vi "Read Status.vi"(6 "Selector":T1, 8 "error in":errorcluster, 11 "MiniIO in":refnum<class "MiniIO.lvclass">) -> (0 "error out":errorcluster, 3 "MiniIO out":refnum<class "MiniIO.lvclass">)   [LabVIEW 2018, in "MiniIO.lvlib" / "MiniIO.lvclass"]
uses:
  MiniIO.lvclass
  PPLs/PLC/Parent/PLC.lvlibp/Custom Controls/Selector.ctl
  PPLs/PLC/Parent/PLC.lvlibp/PLC.lvclass
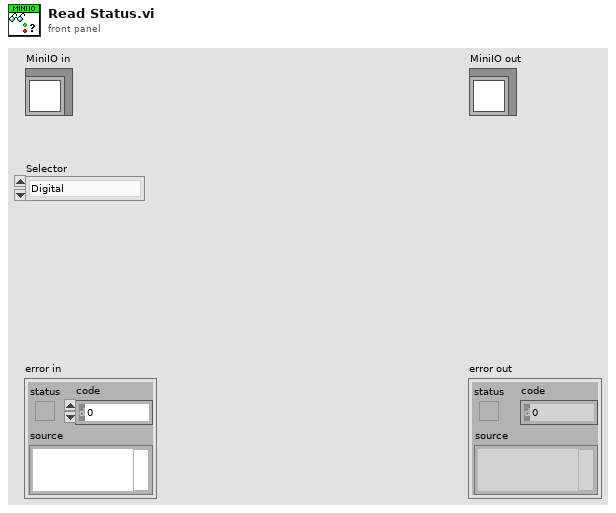
[diagram p1: front panel]
types:
  T1 = typedef "PLC.lvlibp/PLC.lvclass/Selector.ctl" = enum16{"Digital", "Analog"}
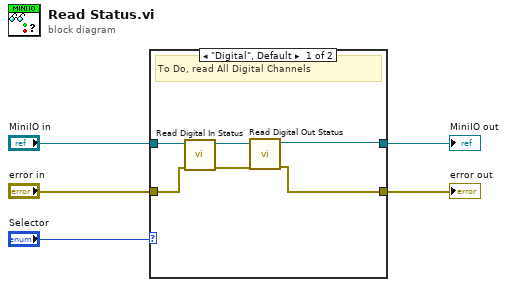
[diagram p0: block diagram]
diagram:
  n1 = case shown="\"Digital\", Default" "Selector" {
    tunnel: "MiniIO in" -> [w11 w13]
    tunnel: [w7 w13] -> w3
    tunnel: "error in" -> [w10 w12]
    tunnel: [w6 w12] -> w1
    frame "Digital", Default {
      # "To Do, read All Digital Channels"
      n2 = call "Read Digital In Status.vi"("error in"=w10, "MiniIO in"=w11) -> ("error out"=w9:errorcluster, "MiniIO out"=w8:refnum<class "MiniIO.lvclass">)  [unwired: 8 in]
      n3 = call "Read Digital Out Status.vi"("error in"=w9, "MiniIO in"=w8) -> ("error out"=w6:errorcluster, "MiniIO out"=w7:refnum<class "MiniIO.lvclass">)  [unwired: 8 in]
    }
    frame "Analog" {
      # "Mini IO does not have Analog"
    }
  }
  "error out" <- w1
  "MiniIO out" <- w3
